vi "Create_Piezo.vi"() -> (0 "Cancel Button Out":bool, 3 "Layer Data Out":T2[](array[typedef]))   [LabVIEW 2022 SP3]
uses:
  Custom_Piezo.ctl
  PZT type.ctl
panel:
  out "Current Layer":i32
  in  "Type":T1
  in  "OK Button":bool
  in  "Dielectric Strength (d31)":dbl
  in  "Thickness":dbl
  in  "Poissoin's Ratio":dbl
  in  "Density":dbl
  in  "Radius":dbl
  in  "Young's Modulus":dbl
  in  "Next Layer":bool
  in  "Cancel Button":bool
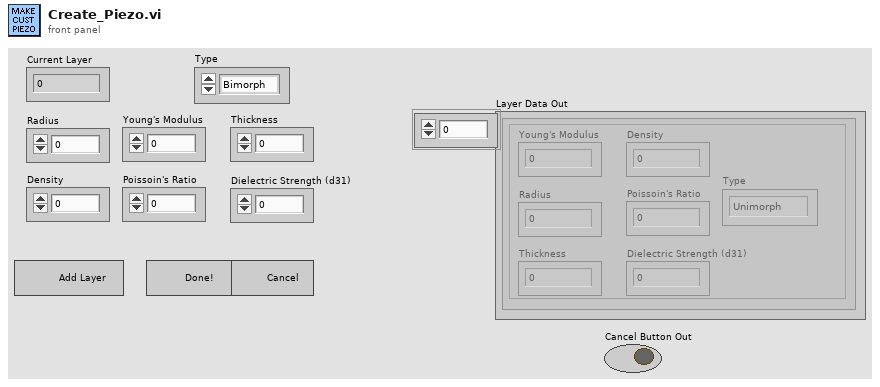
[diagram p1: front panel]
types:
  T1 = typedef "PZT type.ctl" = enum16{"Bimorph", "Unimorph"}
  T2 = typedef "Custom_Piezo.ctl" = cluster{"Young's Modulus":dbl, "Radius":dbl, "Density":dbl, "Poissoin's Ratio":dbl, "Thickness":dbl, "Dielectric Strength (d31)":dbl, "Type":T1}
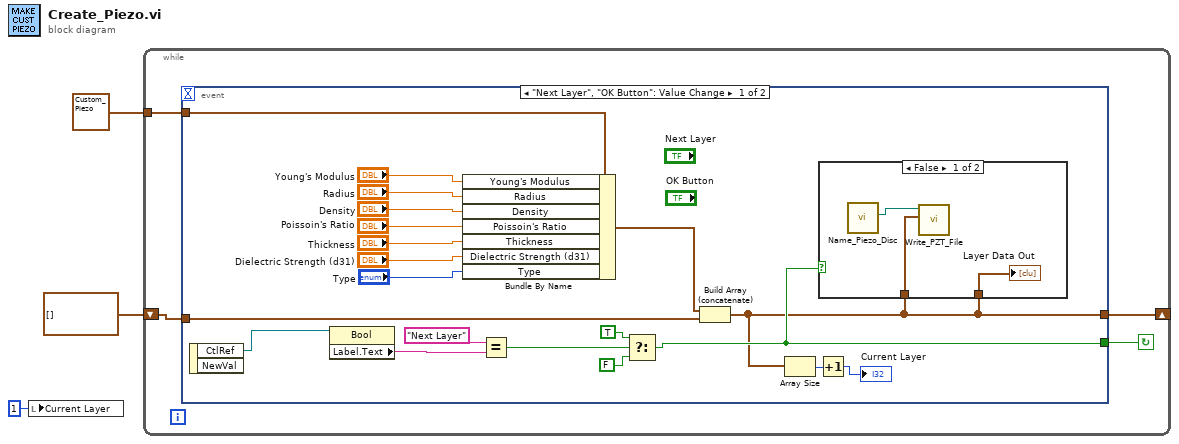
[diagram p0: block diagram]
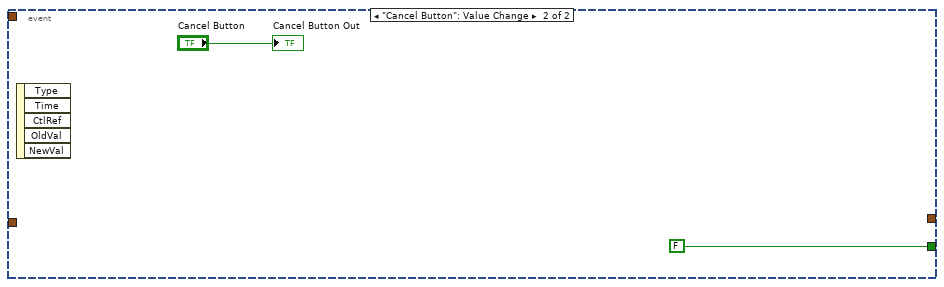
[diagram p3: hidden frame]
diagram:
  n1 = local write "Current Layer"(1 ("Current Layer")) -> ()
  n2 = while {
    tunnel: T2 {"Young's Modulus"=0.0, "Radius"=0.0, "Density"=0.0, "Poissoin's Ratio"=0.0, "Thickness"=0.0, "Dielectric Strength (d31)"=0.0, "Type"=enum."Unimorph"} ("Custom Piezo") -> [w6]
    shift-right: [w5] -> _
    shift-left: T2[] [] -> [w4]
    stop <- w7 continue-if-true
    n3 = event shown="[0] \"Next Layer\", \"OK Button\": Value Change" {
      selector: _ -> [_ _]
      dyn-events: _ -> [_ _]
      timeout: _ -> [_ _]
      tunnel: [w12 FALSE] -> w7
      tunnel: w6 -> [w27 _]
      tunnel: [w10 _] -> w5
      tunnel: w4 -> [w26 _]
      event "Next Layer", "OK Button": Value Change {
        n4 = event-data() -> ("CtlRef"=w18:refnum<vi>)  [unwired: 1 in, 1 out]
        n5 = property class="Bool"(reference=w18) -> ("Label.Text"=w17:string)  [unwired: 1 in, 2 out]
        n6 = Bundle By Name(cluster=w27, "Young's Modulus"="Young's Modulus", "Radius"="Radius", "Density"="Density", "Poissoin's Ratio"="Poissoin's Ratio", "Thickness"="Thickness", "Dielectric Strength (d31)"="Dielectric Strength (d31)", "Type"="Type") -> (w25:T2)
        n7 = Equal?(x="Next Layer", y=w17) -> (x = y?=w15:bool)
        n8 = Select(t=TRUE, s=w15, f=FALSE) -> (s? t:f=w12:bool)
        n9 = Build Array (concatenate)(w25, w26) -> (w10:T2[])
        n10 = Array Size(array=w10) -> (size(s)=w9:i32)
        n11 = Increment(x=w9) -> (x+1=→"Current Layer":i32)
        n12 = case shown="False" w12 {
          tunnel: w10 -> [w30 _]
          tunnel: w10 -> [w28 _]
          frame False {
            n13 = call "Name_Piezo_Disc.vi"() -> ("PZT path out"=w29:path)  [unwired: 11 in]
            n14 = call "Write_PZT_File.vi"("Layer Data"=w28, "PZT filename"=w29) -> ()  [unwired: 9 in, 1 out]
            "Layer Data Out" <- w30
          }
          frame True {
          }
        }
      }
      event "Cancel Button": Value Change {
        n15 = event-data() -> ()  [unwired: 1 in, 5 out]
        "Cancel Button Out" <- "Cancel Button"
      }
    }
  }
